vi "testCommunication.vi"(7 "error in":errorcluster, 10 "RequestData":T2) -> (0 "error out":errorcluster, 2 "Parse Errors":string, 3 "Response Data":T1)   [LabVIEW 2023, in "MES.lvlib"]
uses:
  MES.lvlib
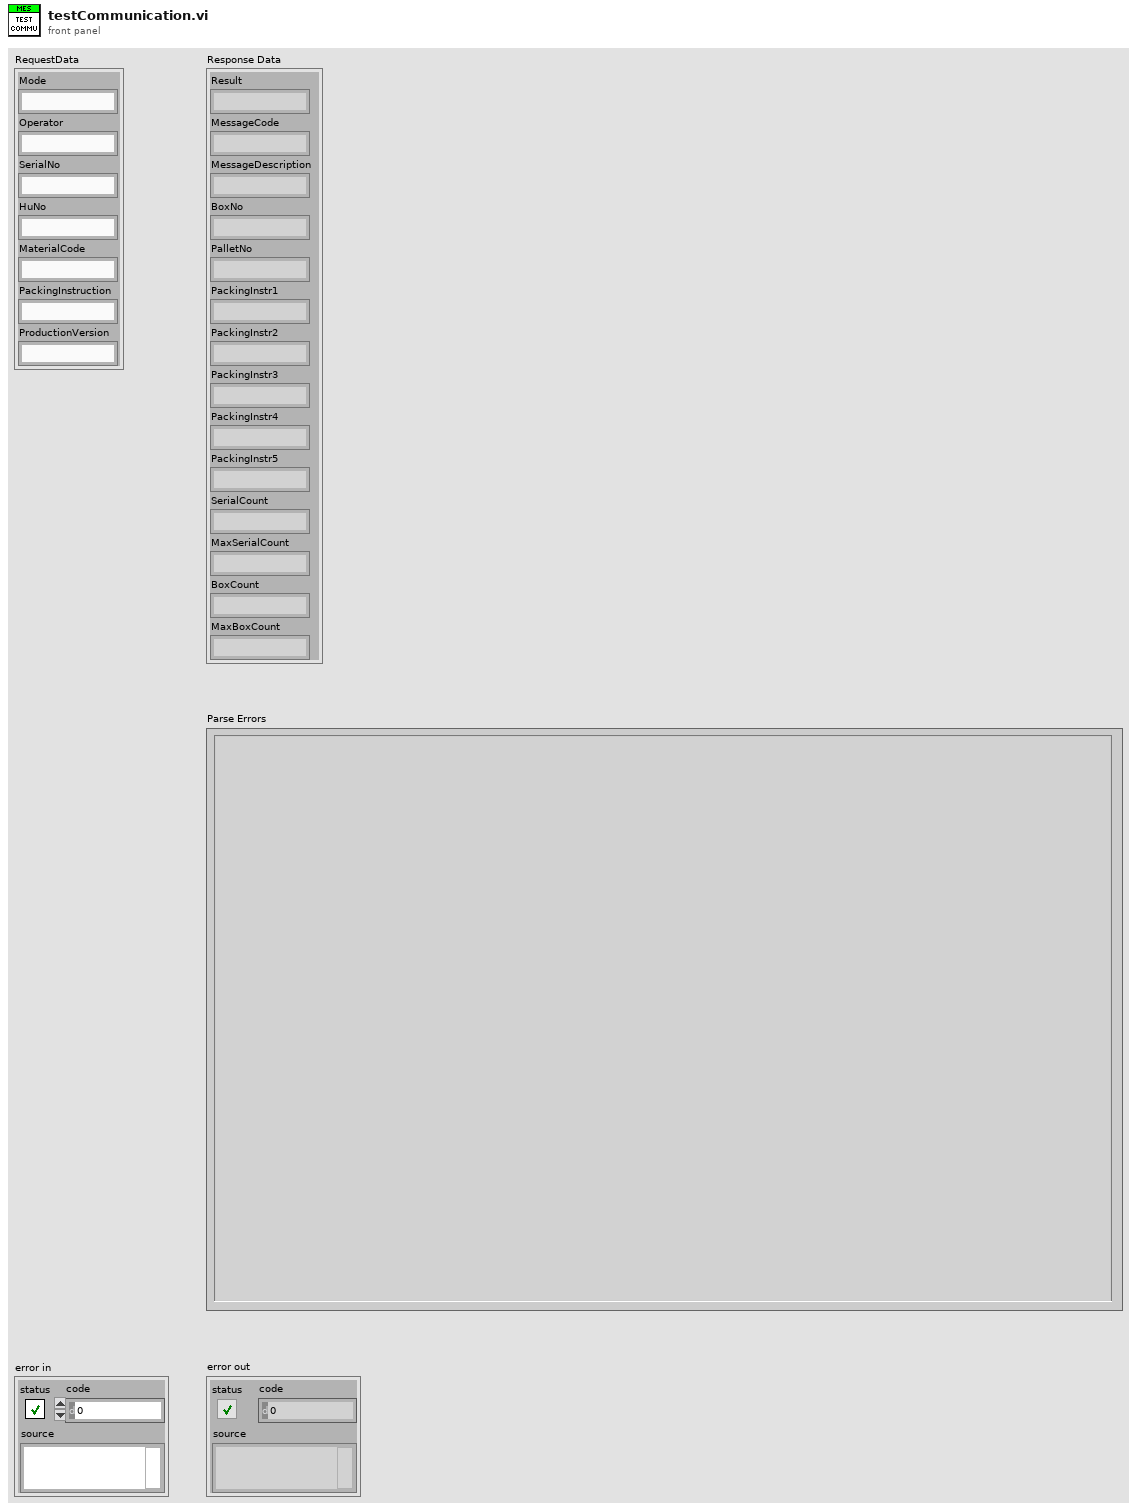
[diagram p1: front panel]
types:
  T1 = cluster{"Result":string, "MessageCode":string, "MessageDescription":string, "BoxNo":string, "PalletNo":string, "PackingInstr1":string, "PackingInstr2":string, "PackingInstr3":string, "PackingInstr4":string, "PackingInstr5":string, "SerialCount":string, "MaxSerialCount":string, "BoxCount":string, "MaxBoxCount":string}
  T2 = cluster{"Mode":string, "Operator":string, "SerialNo":string, "HuNo":string, "MaterialCode":string, "PackingInstruction":string, "ProductionVersion":string}
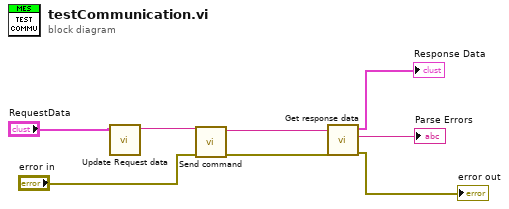
[diagram p0: block diagram]
diagram:
  n1 = call "Update Request data.vi"("RequestData"="RequestData") -> ("RequestXML"=w7:string)  [unwired: 9 in]
  n2 = call "Send command.vi"("error in"="error in", "MES Request"=w7) -> ("error out"=w3:errorcluster, "MES Response"=w4:string)  [unwired: 7 in]
  n3 = call "Get response data.vi"("error in"=w3, "MES Response"=w4) -> ("error out"=→"error out":errorcluster, "Parse Errors"=→"Parse Errors":string, "Response Data"=→"Response Data":T1)  [unwired: 6 in]
